vi "Pump Status.vi"(8 "error in (no error)":errorcluster, 11 "KNF Settings In":T2={"VISA resource name"="", "Simulated?"=TRUE}) -> (0 "error out":errorcluster, 1 "Connection Error":bool, 2 "Pump On?":enum16{"Off", "On", "Not Initialized"}(ring), 3 "KNF Settings Out":T2={"VISA resource name"="", "Simulated?"=TRUE})   [LabVIEW 2018, in "KNF SIMDOS.lvlib"]
uses:
  KNF SIMDOS.lvlib
  Settings Cluster plus SIMDOS.ctl
  <vilib>/KNF LAB/Driver S/Lvlib/SIMLAB_driver_lvclass/StatusRequestMode.ctl
  <vilib>/KNF LAB/Driver S/Lvlib/SIMLAB_driver_lvclass/SIMLAB_driver.lvclass
panel:
  out "PumpStatus":T1 caption="Pump Status"
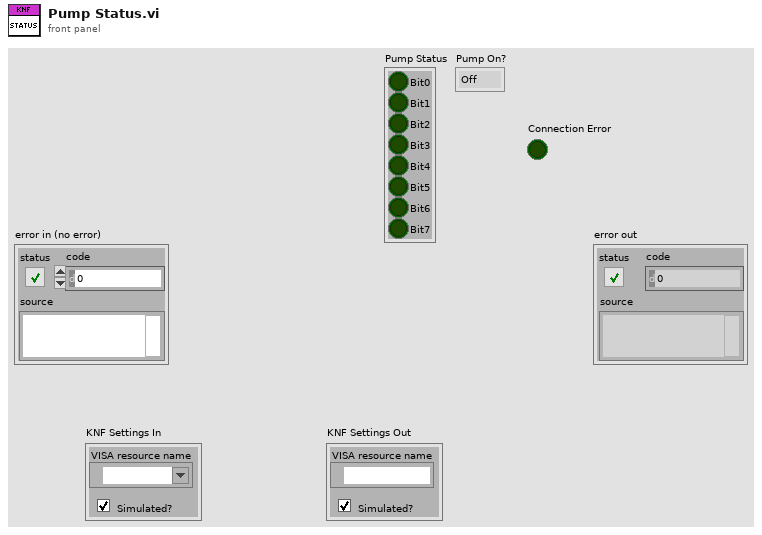
[diagram p1: front panel]
types:
  T1 = cluster{"Bit0":bool, "Bit1":bool, "Bit2":bool, "Bit3":bool, "Bit4":bool, "Bit5":bool, "Bit6":bool, "Bit7":bool}
  T2 = typedef "KNF SIMDOS.lvlib/Settings Cluster plus SIMDOS.ctl" = cluster{"VISA resource name":refnum<visa-resource-name>, "Simulated?":bool}
  T3 = typedef "SIMLAB_driver.lvlib/SIMLAB_driver.lvclass/StatusRequestMode.ctl" = u16
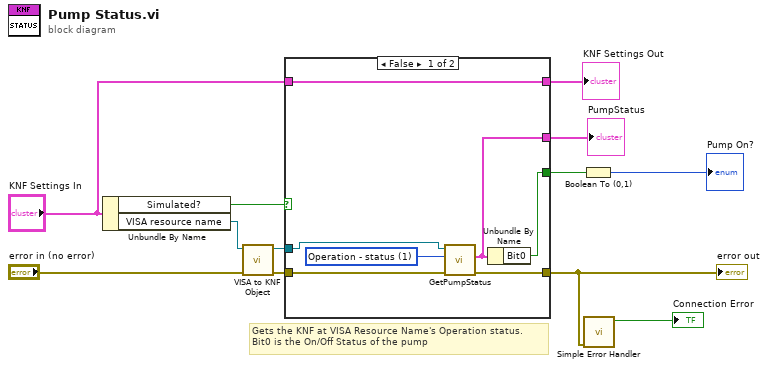
[diagram p0: block diagram]
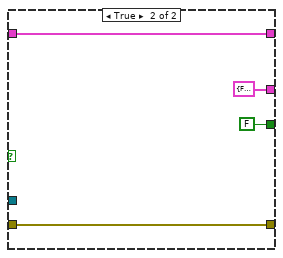
[diagram p2: hidden frame]
diagram:
  # "Gets the KNF at VISA Resource Name's Operation status.\nBit0 is the On/Off Status of the pump"
  n1 = Unbundle By Name("KNF Settings In") -> ("Simulated?"=w12:bool, "VISA resource name"=w4:refnum<visa-resource-name>)
  n2 = call "VISA to KNF Object.vi"("error in (no error)"="error in (no error)", "VISA resource name"=w4) -> ("error out"=w6:errorcluster, "SIMDOS out"=w5:refnum<class "SIMLAB_driver.lvclass">)  [unwired: 8 in]
  n3 = case shown="False" w12 {
    tunnel: [w14 w23] -> w11
    tunnel: "KNF Settings In" -> [w14 w23]
    tunnel: [w17 w22] -> w9
    tunnel: w6 -> [w16 w22]
    tunnel: w5 -> [w15 _]
    tunnel: [w18 FALSE] -> w3
    tunnel: [w13 T1 {"Bit0"=FALSE, "Bit1"=FALSE, "Bit2"=FALSE, "Bit3"=FALSE, "Bit4"=FALSE, "Bit5"=FALSE, "Bit6"=FALSE, "Bit7"=FALSE} ("PumpStatus")] -> w1
    frame False {
      w19 = T3 1 items=["Operation - status"=1, "System - status"=2, "Run mode - status"=3, "Dispense mode - status"=4, "Reserved"=5, "Fault diagnosis"=6] ("StatusRequestMode")
      n4 = call <vilib>:"GetPumpStatus.vi"("error in (no error)"=w16, "StatusRequestMode"=w19, "SIMDOS in"=w15) -> ("error out"=w17:errorcluster, "PumpStatus"=w13:T1)  [unwired: 6 in, 1 out]
      n5 = Unbundle By Name(w13) -> ("Bit0"=w18:bool)
    }
    frame True {
    }
  }
  "error out" <- w9
  "KNF Settings Out" <- w11
  "PumpStatus" <- w1
  n6 = Boolean To (0,1)(Boolean=w3) -> (0, 1=→"Pump On?":i16)
  n7 = call <vilib>:"Simple Error Handler.vi"("error in (no error)"=w9) -> ("error?"=→"Connection Error":bool)  [unwired: 4 in, 4 out]
